vi "Advanced Connection Settings Dialog.vi"(8 "Error In":errorcluster) -> (0 "Error Out":errorcluster)   [LabVIEW 2014]
doc: "Provides Connection Settings with reading and writing to xml file"
uses:
  Controls/Advanced Connection Settings Cluster.ctl
  Controls/Configuration Files.ctl
  Convert From XML Configuration Files - Polymorphic/Advanced Connection Settings Polymporhic.vi
panel:
  in  "Cancel Button":bool
  in  "OK Button":bool
  in  "Advanced Connection Settings Cluster":T1={"Baud Rate"=0, "Data Bits"=8, "Parity"=0, "Stop Bits"=10, "Flow Control"=0, "Termination Char"=0, "Enable Termination Char"=FALSE} {"Flow Control" items=["None", "XON/XOFF", "RTS/CTS", "XON/XOFF & RTS/CTS", "DTR/DSR", "XON/XOFF & DTR/DSR"]; "Stop Bits" items=["1.0"=10, "1.5"=15, "2.0"=20]; "Parity" items=["None", "Odd", "Even", "Mark", "Space"]; "Baud Rate" items=["100"=100, "300"=300, "600"=600, "1200"=1200, "2400"=2400, "4800"=4800, "9600"=9600, "14400"=14000, "19200"=19200, "28800"=28800, "38400"=38400, "56000"=56000, "57600"=57600, "115200"=13]}
  # "ADVANCED CONNECTION SETTINGS"
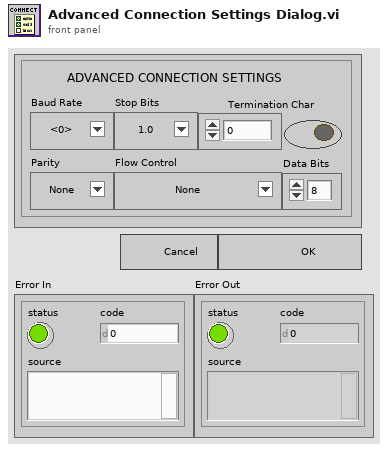
[diagram p1: front panel]
types:
  T1 = typedef "Advanced Connection Settings Cluster.ctl" = cluster{"Baud Rate":u32, "Data Bits":u16, "Parity":u16, "Stop Bits":u16, "Flow Control":u16, "Termination Char":u8, "Enable Termination Char":bool}
  T2 = typedef "Configuration Files.ctl" = string
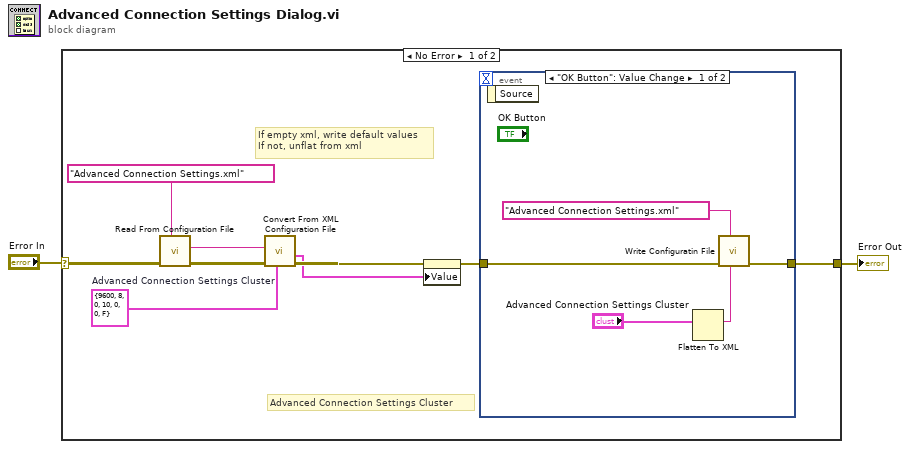
[diagram p0: block diagram]
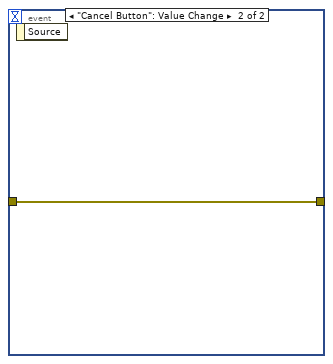
[diagram p2: hidden frame]
diagram:
  n1 = case shown="No Error" "Error In" {
    selector: "Error In" -> [w9 w18]
    tunnel: [w11 w18] -> w1
    frame No Error {
      w6 = T1 {"Baud Rate"=9600, "Data Bits"=8, "Parity"=0, "Stop Bits"=10, "Flow Control"=0, "Termination Char"=0, "Enable Termination Char"=FALSE}  # Advanced Connection Settings Cluster
      # "If empty xml, write default values\nIf not, unflat from xml"
      # "Advanced Connection Settings Cluster"
      n2 = call "Read From Configuration File.vi"("Settings"=T2 "Advanced Connection Settings.xml", "error in (no error)"=w9) -> ("error out"=w7:errorcluster, "XML Elements"=w5:string)  [unwired: 8 in]
      n3 = call-poly "Convert From XML Configuration File.vi"("Advanced Connection Settings Cluster In"=w6, "error in (no error)"=w7, "XML Elements"=w5) -> ("error out"=w4:errorcluster, "Advanced Connection Settings Cluster Out"=w3:T1)  [unwired: 7 in]
      n4 = property on="Advanced Connection Settings Cluster" class="Clust (strict)"(error in=w4, "Value"=w3) -> (error out=w10:errorcluster)  [unwired: 1 in, 1 out]
      n5 = event shown="[0] \"OK Button\": Value Change" {
        selector: _ -> [_ _]
        dyn-events: _ -> [_ _]
        timeout: _ -> [_ _]
        tunnel: w10 -> [w16 w17]
        tunnel: [w14 w17] -> w11
        event "OK Button": Value Change {
          n6 = event-data() -> ()  [unwired: 1 in, 1 out]
          n7 = Flatten To XML(anything="Advanced Connection Settings Cluster") -> (xml string=w12:string)
          n8 = call "Write Configuratin File.vi"("XML String"=w12, "Settings"=T2 "Advanced Connection Settings.xml", "error in (no error)"=w16) -> ("error out"=w14:errorcluster)  [unwired: 8 in]
        }
        event "Cancel Button": Value Change {
          n9 = event-data() -> ()  [unwired: 1 in, 1 out]
        }
      }
    }
    frame Error {
    }
  }
  "Error Out" <- w1
